vi "gradient_ascent_test_2d.vi"() -> ()   [LabVIEW 2024]
uses:
  <vilib>/Math Plots/3D Math Plots/3D Scatter/3D Scatter XCtrl/3D Scatter.xctl
  <vilib>/Math Plots/3D Math Plots/3D Scatter/3D Scatter Datatype/Public/Plot Helper (Vector).vi
  <vilib>/Math Plots/3D Math Plots/3D Scatter/3D Scatter Datatype/3D Scatter Datatype.lvclass
panel:
  out "Array":dbl[][](array[numeric])
  out "3D Scatter":refnum<class "3D Plot Datatype.lvclass">[](xcontrol)
  out "Intensity Graph":dbl[][](graph)
  out "diff":dbl[](array[numeric])
  out "end result":dbl[](array[numeric])
  in  "k":dbl=-25.0
  out "start X":dbl[](array[numeric])
  out "StdDev":dbl[](array[numeric])
  out "Mean":dbl[](array[numeric])
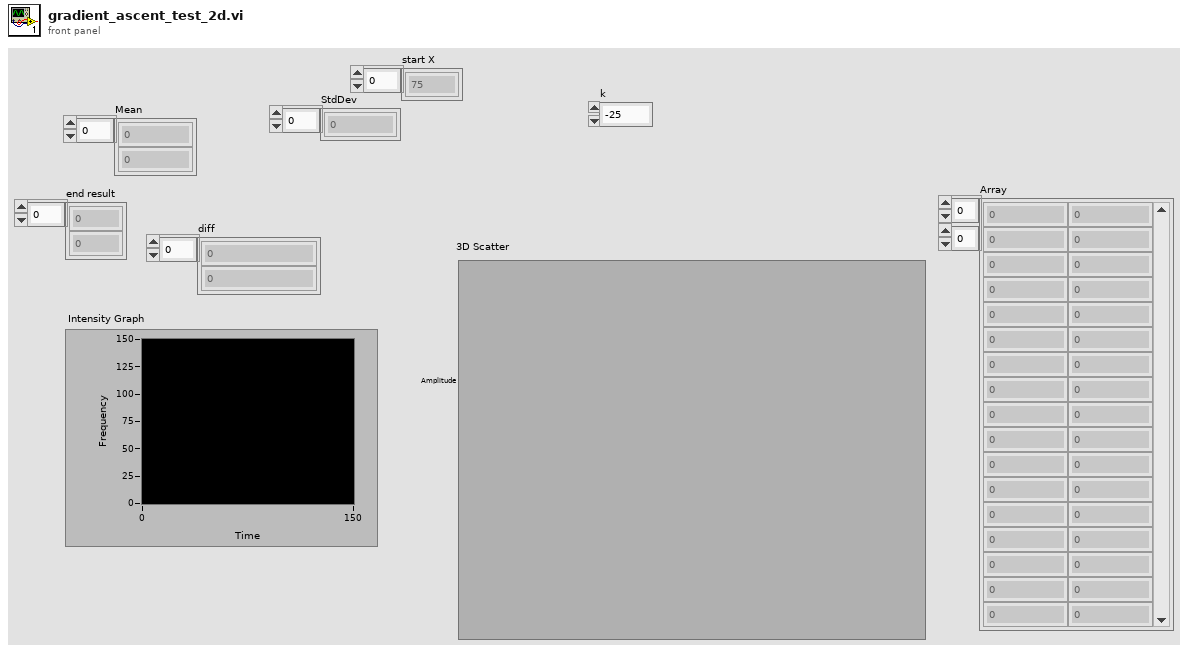
[diagram p1: front panel]
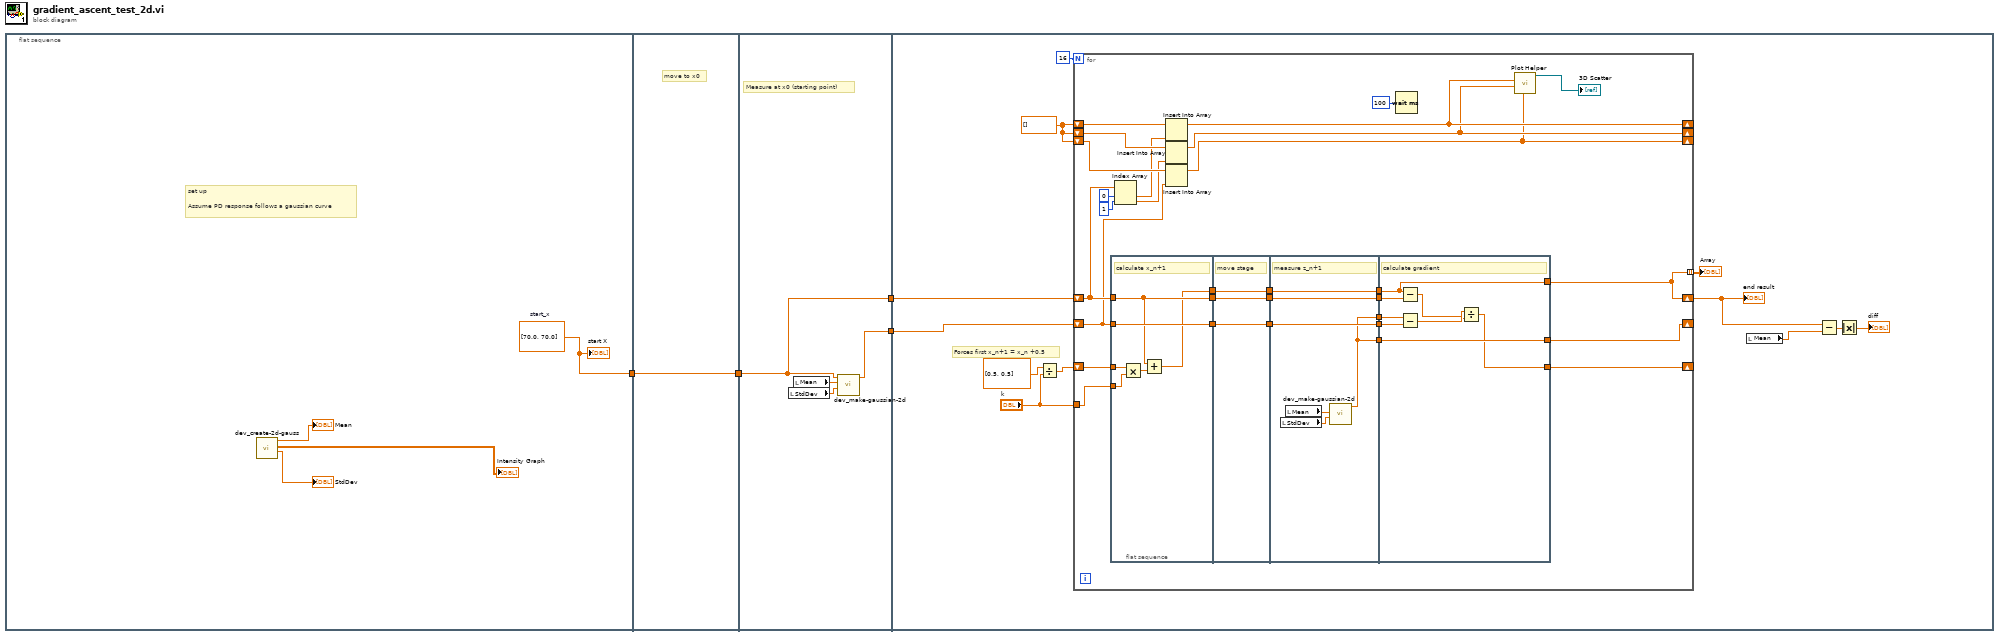
[diagram p0: block diagram]
diagram:
  n1 = flat-sequence {
    tunnel: [w8] -> w4
    tunnel: w4 -> [w9]
    tunnel: [w9] -> w3
    tunnel: w3 -> [w11]
    tunnel: [w11] -> w2
    tunnel: [w10] -> w1
    tunnel: w1 -> [w23]
    tunnel: w2 -> [w24]
    frame #0 {
      w8 = dbl[] [70.0, 70.0]  # start_x
      # "set up\n\nAssume PD response follows a gaussian curve"
      n2 = call "dev_create-2d-gauss.vi"() -> ("StdDev"=→"StdDev":dbl[], "Intensity Graph"=→"Intensity Graph":dbl[][], "Mean"=→"Mean":dbl[])  [unwired: 9 in]
      "start X" <- w8
    }
    frame #1 {
      # "move to x0"
    }
    frame #2 {
      # "Measure at x0 (starting point)"
      n3 = local read "StdDev"() -> (w12:dbl[])
      n4 = local read "Mean"() -> (w13:dbl[])
      n5 = call "dev_make-gaussian-2d.vi"("StdDev"=w12, "Mean"=w13, "in"=w11) -> ("out"=w10:dbl)  [unwired: 8 in]
    }
    frame #3 {
      w15 = dbl[] []
      # "Forces first x_n+1 = x_n +0.5"
      n6 = Divide(x=dbl[] [0.5, 0.5], y="k") -> (x/y=w17:dbl[])
      n7 = for {
        N: 16 -> [_]
        shift-right: [w26] -> _
        shift-left: w17 -> [w46]
        shift-right: [w29] -> w22
        shift-left: w24 -> [w44]
        shift-right: [w27] -> _
        shift-left: w23 -> [w43]
        tunnel: "k" -> [w45]
        shift-right: [w40] -> _
        shift-left: w15 -> [w51]
        shift-right: [w41] -> _
        shift-left: w15 -> [w52]
        shift-right: [w42] -> _
        shift-left: w15 -> [w53]
        tunnel: [w29] -> w14 mode=indexing
        n8 = flat-sequence {
          tunnel: w46 -> [w60]
          tunnel: w45 -> [w59]
          tunnel: w44 -> [w57]
          tunnel: w43 -> [w61]
          tunnel: [w57] -> w37
          tunnel: [w61] -> w34
          tunnel: [w56] -> w31
          tunnel: [w64] -> w38
          tunnel: w37 -> [w64]
          tunnel: [w63] -> w35
          tunnel: w34 -> [w63]
          tunnel: [w62] -> w32
          tunnel: w31 -> [w62]
          tunnel: [w68] -> w39
          tunnel: w38 -> [w68]
          tunnel: [w67] -> w36
          tunnel: w35 -> [w67]
          tunnel: [w66] -> w33
          tunnel: w32 -> [w66]
          tunnel: [w65] -> w30
          tunnel: [w65] -> w28
          tunnel: w39 -> [w76]
          tunnel: w36 -> [w77]
          tunnel: w33 -> [w73]
          tunnel: w30 -> [w78]
          tunnel: [w73] -> w29
          tunnel: w28 -> [w72]
          tunnel: [w72] -> w27
          tunnel: [w71] -> w26
          frame #0 {
            # "calculate x_n+1"
            n9 = Multiply(x=w60, y=w59) -> (x*y=w58:dbl[])
            n10 = Add(x=w57, y=w58) -> (x+y=w56:dbl[])
          }
          frame #1 {
            # "move stage"
          }
          frame #2 {
            # "measure z_n+1"
            n11 = local read "StdDev"() -> (w69:dbl[])
            n12 = local read "Mean"() -> (w70:dbl[])
            n13 = call "dev_make-gaussian-2d.vi"("StdDev"=w69, "Mean"=w70) -> ("out"=w65:dbl)  [unwired: 9 in]
          }
          frame #3 {
            # "calculate gradient"
            n14 = Subtract(x=w73, y=w76) -> (x-y=w74:dbl[])
            n15 = Subtract(x=w78, y=w77) -> (x-y=w75:dbl)
            n16 = Divide(x=w75, y=w74) -> (x/y=w71:dbl[])
          }
        }
        n17 = Index Array(array=w44, index #1=0 ("index"), index #2=1 ("index")) -> (element #1=w50:dbl, element #2=w49:dbl)
        n18 = Insert Into Array(array=w53, new element=w50) -> (w42:dbl[])  [unwired: 1 in]
        n19 = Insert Into Array(array=w52, new element=w49) -> (w41:dbl[])  [unwired: 1 in]
        n20 = Insert Into Array(array=w51, new element=w43) -> (w40:dbl[])  [unwired: 1 in]
        n21 = Wait (ms)(milliseconds to wait=u32 100) -> ()  [unwired: 1 out]
        n22 = call-poly <vilib>:"Plot Helper.vi"("z vector"=w40, "y vector"=w41, "x vector"=w42) -> ("3D Plot lvclass Array out"=→"3D Scatter":refnum<class "3D Plot Datatype.lvclass">[])  [unwired: 3 in, 5 out]
      }
      "end result" <- w22
      "Array" <- w14
      n23 = local read "Mean"() -> (w21:dbl[])
      n24 = Subtract(x=w22, y=w21) -> (x-y=w20:dbl[])
      n25 = Absolute Value(x=w20) -> (abs(x)=→"diff":dbl[])
    }
  }
